vi "Auto Loop 0.vi"(2 "Auto State":u8, 3 "Call Context":T1) -> (0 "Loop 0 Data":T2, 1 "SubState 0":T3=enum."driver control")   [LabVIEW 2013]
uses:
  typedefs/State Machine/subStates.ctl
  typedefs/Loop Datatypes/Loop 0 Datatype.ctl
  <vilib>/Rock Robotics/WPI/DriverStation/WPI_DriverStationDerivedRobotMode.ctl
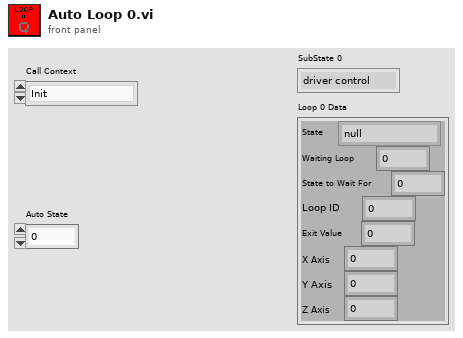
[diagram p1: front panel]
types:
  T1 = typedef "WPI_DriverStationDerivedRobotMode.ctl" = enum16{"Init", "Execute", "Stop"}
  T2 = typedef "Loop 0 Datatype.ctl" = cluster{"State":T3, "Waiting Loop":i32, "State to Wait For":i32, "Loop ID":i32, "Exit Value":i32, "X Axis":dbl, "Y Axis":dbl, "Z Axis":dbl}
  T3 = typedef "subStates.ctl" = enum16{"null", "wait", "driver control", "auto", "manual override", "hold position", "rotate", "pickup", "pass", "load", "goto shoot", "shoot high goal", "shoot low goal", "cancel arm", "cancel shooter", "end", "test"}
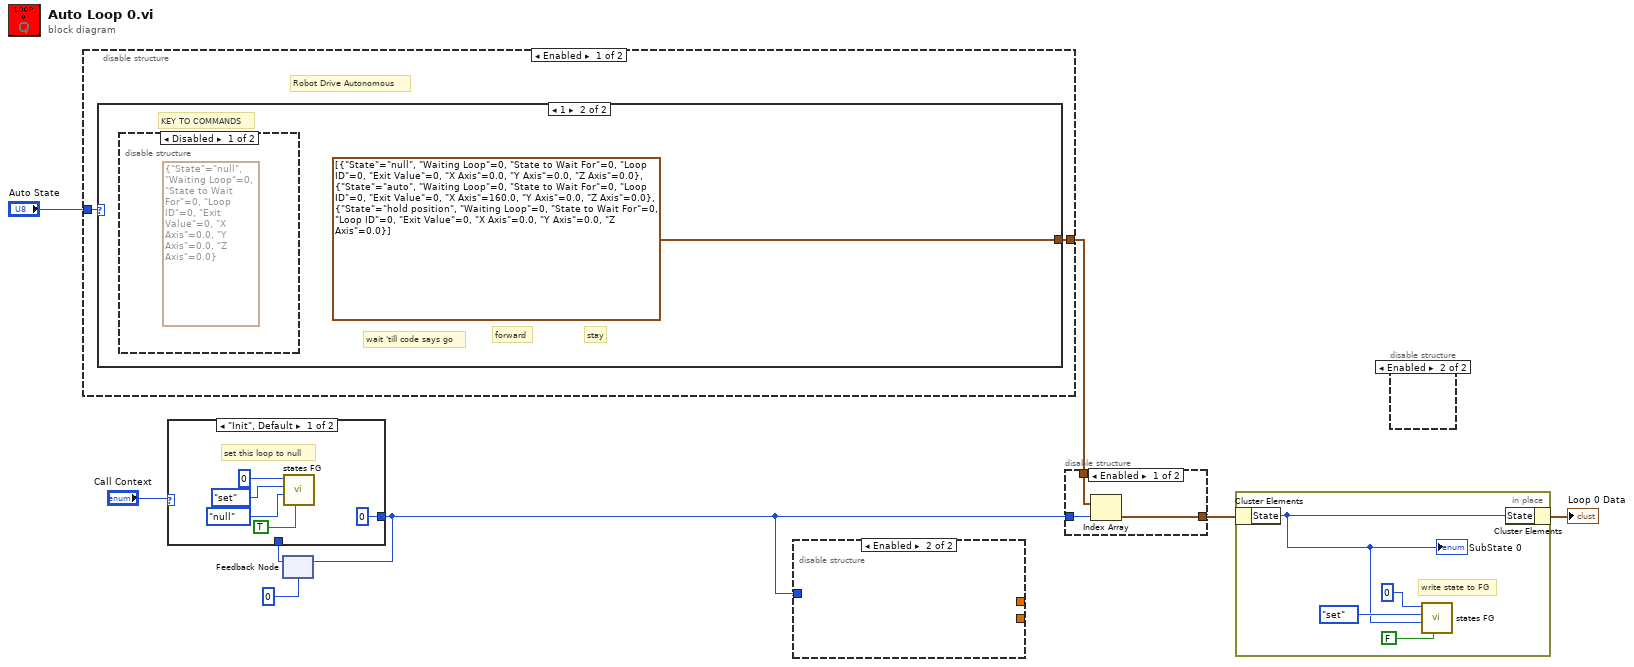
[diagram p0: block diagram]
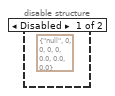
[diagram p2: hidden frame]
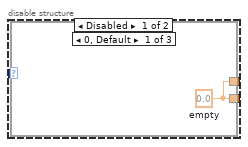
[diagram p3: hidden frame]
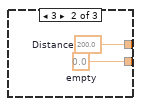
[diagram p4: hidden frame]
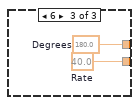
[diagram p5: hidden frame]
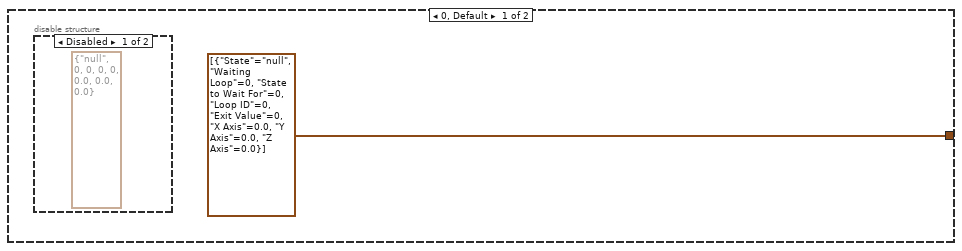
[diagram p7: hidden frame]
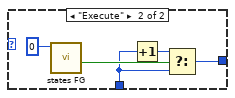
[diagram p11: hidden frame]
diagram:
  n1 = disable-structure shown="Enabled" {
    disable-tunnel: "Auto State" -> [w10 _]
    disable-tunnel: [w9 _] -> w5
    frame Enabled {
      # "Robot Drive Autonomous"
      n2 = case shown="1" w10 {
        tunnel: [T2[] [{"State"=enum."null", "Waiting Loop"=0, "State to Wait For"=0, "Loop ID"=0, "Exit Value"=0, "X Axis"=0.0, "Y Axis"=0.0, "Z Axis"=0.0}] T2[] [{"State"=enum."null", "Waiting Loop"=0, "State to Wait For"=0, "Loop ID"=0, "Exit Value"=0, "X Axis"=0.0, "Y Axis"=0.0, "Z Axis"=0.0}, {"State"=enum."auto", "Waiting Loop"=0, "State to Wait For"=0, "Loop ID"=0, "Exit Value"=0, "X Axis"=160.0, "Y Axis"=0.0, "Z Axis"=0.0}, {"State"=enum."hold position", "Waiting Loop"=0, "State to Wait For"=0, "Loop ID"=0, "Exit Value"=0, "X Axis"=0.0, "Y Axis"=0.0, "Z Axis"=0.0}]] -> w9
        frame 0, Default {
          n3 = disable-structure shown="Disabled" {
            frame Disabled {
              (unwired) T2 {"State"=enum."null", "Waiting Loop"=0, "State to Wait For"=0, "Loop ID"=0, "Exit Value"=0, "X Axis"=0.0, "Y Axis"=0.0, "Z Axis"=0.0} ("Loop 0 Data")
            }
            frame Enabled {
            }
          }
        }
        frame 1 {
          # "wait 'till code says go"
          # "stay"
          # "forward"
          # "KEY TO COMMANDS"
          n4 = disable-structure shown="Disabled" {
            frame Disabled {
              (unwired) T2 {"State"=enum."null", "Waiting Loop"=0, "State to Wait For"=0, "Loop ID"=0, "Exit Value"=0, "X Axis"=0.0, "Y Axis"=0.0, "Z Axis"=0.0} ("Loop 0 Data")
            }
            frame Enabled {
            }
          }
        }
      }
    }
    frame Disabled {
    }
  }
  n5 = feedback #1(0) -> (w6:i32)
  n6 = case shown="\"Init\", Default" "Call Context" {
    tunnel: w6 -> [_ w19]
    tunnel: [0 ("subState out") w21] -> w4
    frame "Init", Default {
      # "set this loop to null"
      n7 = call "states FG.vi"("exit in"=TRUE, "subState in"=subStates."null", "menu (get)"=enum16{"set", "get"}."set", "Loop ID"=0) -> ()  [unwired: 4 in, 4 out]
    }
    frame "Execute" {
      n8 = call "states FG.vi"("Loop ID"=0) -> ("exit out"=w20:bool)  [unwired: 7 in, 3 out]
      n9 = Increment(x=w19) -> (x+1=w18:i32)
      n10 = Select(t=w18, s=w20, f=w19) -> (s? t:f=w21:i32)
    }
  }
  n11 = feedback-in #1(w4) -> ()
  n12 = disable-structure shown="Enabled" {
    disable-tunnel: [w25 _] -> _
    disable-tunnel: w4 -> [w24 _]
    disable-tunnel: [w23 _] -> _
    frame Disabled {
      n13 = case shown="0, Default" w24 {
        tunnel: [w26 w28 w30] -> w25
        tunnel: [w26 w27 w29] -> w23
        frame 0, Default {
          w26 = 0.0  # empty
        }
        frame 3 {
          w27 = 0.0  # empty
          w28 = 200.0  # Distance
        }
        frame 6 {
          w29 = 40.0  # Rate
          w30 = 180.0  # Degrees
        }
      }
    }
    frame Enabled {
    }
  }
  n14 = disable-structure shown="Enabled" {
    disable-tunnel: w5 -> [w33 _]
    disable-tunnel: w4 -> [w32 _]
    disable-tunnel: [w31 _] -> w3
    frame Enabled {
      n15 = Index Array(array=w33, index=w32) -> (element=w31:T2)
    }
    frame Disabled {
    }
  }
  n16 = in-place {
    # "write state to FG"
    n17 = in-place-cluster #2(w3) -> ("State"=w34:T3)
    "SubState 0" <- w34
    n18 = call "states FG.vi"("exit in"=FALSE, "subState in"=w34, "menu (get)"=enum16{"set", "get"}."set", "Loop ID"=0) -> ()  [unwired: 4 in, 4 out]
    n19 = in-place-cluster #2("State"=w34) -> (→"Loop 0 Data":T2)
  }
  n20 = disable-structure shown="Enabled" {
    frame Disabled {
      (unwired) T2 {"State"=enum."null", "Waiting Loop"=0, "State to Wait For"=0, "Loop ID"=0, "Exit Value"=0, "X Axis"=0.0, "Y Axis"=0.0, "Z Axis"=0.0} ("Loop 0 Data 2")
    }
    frame Enabled {
    }
  }
